vi "_Doubles To Base64.vi"(1 "Little Endian (F)":bool, 2 "Doubles":dbl[](array[numeric]) format="%#.6f") -> (0 "Base64 String":string)   [LabVIEW 2012]
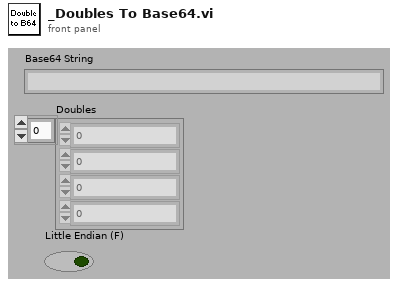
[diagram p1: front panel]
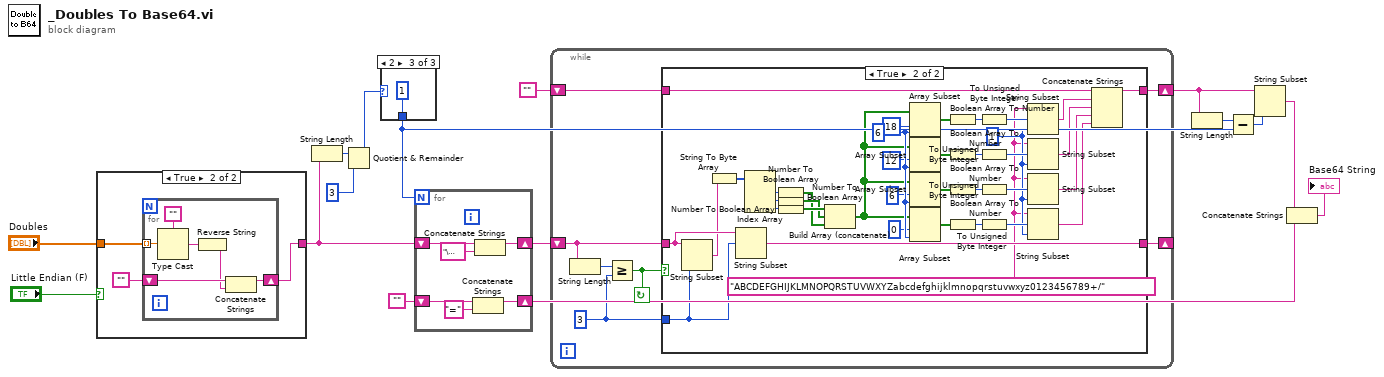
[diagram p0: block diagram]
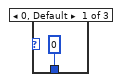
[diagram p2: hidden frame]
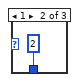
[diagram p3: hidden frame]
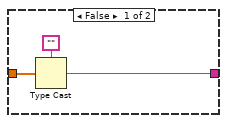
[diagram p5: hidden frame]
diagram:
  n1 = case shown="True" "Little Endian (F)" {
    tunnel: "Doubles" -> [w18 w22]
    tunnel: [w17 w20] -> w12
    frame False {
      n2 = Type Cast(type="", x=w18) -> (*(type *) &x=w17:string)
    }
    frame True {
      n3 = for {
        tunnel: w22 -> [w27] mode=indexing
        shift-right: [w25] -> w20
        shift-left: "" -> [w24]
        n4 = Type Cast(type="", x=w27) -> (*(type *) &x=w26:string)
        n5 = Reverse String(1:w26) -> (0:w23:string)
        n6 = Concatenate Strings(w24, w23) -> (w25:string)
      }
    }
  }
  n7 = String Length(string=w12) -> (length=w14:i32)
  n8 = Quotient & Remainder(x=w14, y=3) -> (x-y*floor(x/y)=w2:i32)  [unwired: 1 out]
  n9 = case shown="2" w2 {
    tunnel: [0 ("y") 2 ("y") 1 ("y")] -> w1
    frame 0, Default {
    }
    frame 1 {
    }
    frame 2 {
    }
  }
  n10 = for {
    N: w1 -> [_]
    shift-right: [w35] -> w11
    shift-left: w12 -> [w37]
    shift-right: [w32] -> w5
    shift-left: "" -> [w33]
    n11 = Concatenate Strings(w33, "=" ("string")) -> (w32:string)
    n12 = Concatenate Strings(w37, "\u0000" ("string")) -> (w35:string)
  }
  n13 = while {
    shift-right: [w41] -> _
    shift-left: w11 -> [w42]
    shift-right: [w38] -> w8
    shift-left: "" -> [w39]
    stop <- w43 continue-if-true
    w40 = 3 ("Precision (32)")
    n14 = String Length(string=w42) -> (length=w44:i32)
    n15 = Greater Or Equal?(x=w44, y=w40) -> (x >= y?=w43:bool)
    n16 = case shown="True" w43 {
      tunnel: w42 -> [w46 w82]
      tunnel: [w46 w83] -> w41
      tunnel: w40 -> [_ w81]
      tunnel: w39 -> [w45 w80]
      tunnel: [w45 w79] -> w38
      frame False {
      }
      frame True {
        w52 = 1 ("index")
        w51 = "ABCDEFGHIJKLMNOPQRSTUVWXYZabcdefghijklmnopqrstuvwxyz0123456789+/"
        w69 = 6 ("length")
        n17 = String Subset(string=w82, length (rest)=w81) -> (substring=w78:string)  [unwired: 1 out]
        n18 = String To Byte Array(string=w78) -> (unsigned byte array=w77:u8[])
        n19 = String Subset(string=w82, offset (0)=w81) -> (substring=w83:string)  [unwired: 1 out]
        n20 = Index Array(array=w77) -> (element #1=w75:u8, element #2=w74:u8, element #3=w76:u8)  [unwired: 3 in]
        n21 = Number To Boolean Array(number=w75) -> (Boolean array=w70:bool[])
        n22 = Number To Boolean Array(number=w74) -> (Boolean array=w71:bool[])
        n23 = Number To Boolean Array(number=w76) -> (Boolean array=w72:bool[])
        n24 = Build Array (concatenate)(w72, w71, w70) -> (w67:bool[])
        n25 = Array Subset(array=w67, index=18, length=w69) -> (w63:bool[])
        n26 = Array Subset(array=w67, index=12, length=w69) -> (w61:bool[])
        n27 = Array Subset(array=w67, index=6, length=w69) -> (w59:bool[])
        n28 = Array Subset(array=w67, index=0, length=w69) -> (w57:bool[])
        n29 = Boolean Array To Number(Boolean array=w63) -> (number=w64:u8)
        n30 = Boolean Array To Number(Boolean array=w61) -> (number=w62:u8)
        n31 = Boolean Array To Number(Boolean array=w59) -> (number=w60:u8)
        n32 = Boolean Array To Number(Boolean array=w57) -> (number=w58:u8)
        n33 = To Unsigned Byte Integer(number=w64) -> (unsigned 8bit integer=w56:u8)
        n34 = To Unsigned Byte Integer(number=w62) -> (unsigned 8bit integer=w55:u8)
        n35 = To Unsigned Byte Integer(number=w60) -> (unsigned 8bit integer=w54:u8)
        n36 = To Unsigned Byte Integer(number=w58) -> (unsigned 8bit integer=w53:u8)
        n37 = String Subset(string=w51, offset (0)=w56, length (rest)=w52) -> (substring=w50:string)
        n38 = String Subset(string=w51, offset (0)=w55, length (rest)=w52) -> (substring=w49:string)
        n39 = String Subset(string=w51, offset (0)=w54, length (rest)=w52) -> (substring=w48:string)
        n40 = String Subset(string=w51, offset (0)=w53, length (rest)=w52) -> (substring=w47:string)
        n41 = Concatenate Strings(w80, w50, w49, w48, w47) -> (w79:string)
      }
    }
  }
  n42 = String Length(string=w8) -> (length=w9:i32)
  n43 = Subtract(x=w9, y=w1) -> (x-y=w7:i32)
  n44 = String Subset(string=w8, length (rest)=w7) -> (substring=w6:string)  [unwired: 1 out]
  n45 = Concatenate Strings(w6, w5) -> (→"Base64 String":string)
